vi "GetModeAndParameters.vi"(8 "error in (no error)":errorcluster, 10 "Parameters":dbl[](array[numeric])) -> (0 "error out":errorcluster, 2 "Parameters Out":dbl[](array[numeric]), 3 "f":T1=enum."Skip")   [LabVIEW 2017, in "WordManipulationLibrary.lvlib"]
uses:
  WordManipulationLibrary.lvlib
  Mode.ctl
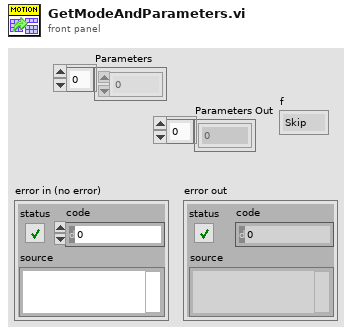
[diagram p1: front panel]
types:
  T1 = typedef "WordManipulationLibrary.lvlib/Mode.ctl" = enum16{"Reserved", "Profile Position Mode", "Velocity Mode", "Profile Velocity Mode", "Profile Torque Mode", "Reserved 2", "Reference Mode", "Interpolated Position Mode", "Skip"}
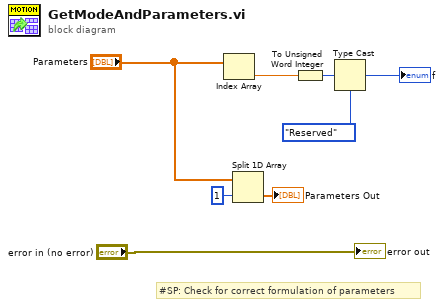
[diagram p0: block diagram]
diagram:
  # "#SP: Check for correct formulation of parameters"
  n1 = Index Array(array="Parameters") -> (element=w7:dbl)  [unwired: 1 in]
  n2 = Split 1D Array(array="Parameters", index=1) -> (second subarray=→"Parameters Out":dbl[])  [unwired: 1 out]
  n3 = To Unsigned Word Integer(number=w7) -> (unsigned 16bit integer=w8:u16)
  n4 = Type Cast(type=Mode."Reserved" ("f"), x=w8) -> (*(type *) &x=→"f":T1)
  "error out" <- "error in (no error)"
